vi "Call Asynchronous.vi"(8 "error in":errorcluster, 10 "Data In":variant, 11 "VI Path":path) -> (0 "error out":errorcluster)   [LabVIEW 2020]
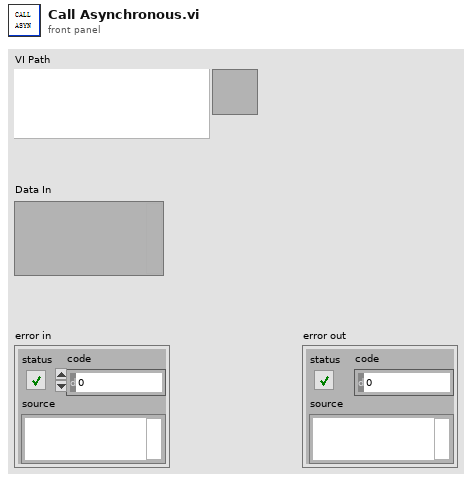
[diagram p1: front panel]
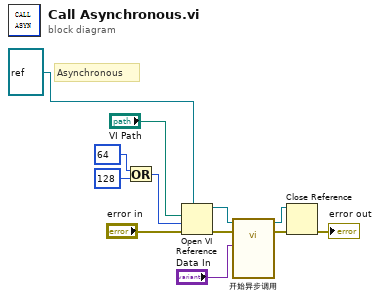
[diagram p0: block diagram]
diagram:
  # "Asynchronous"
  n1 = Or(x=64 ("选项"), y=128 ("选项")) -> (x .or. y?=w12:i32)
  n2 = Open VI Reference(type specifier VI Refnum (for type only)=refnum<vi> refnum, vi path="VI Path", options=w12, error in (no error)="error in") -> (vi reference=w11:refnum<vi>, error out=w10:errorcluster)  [unwired: 2 in]
  n3 = call-by-ref "开始异步调用"(reference=w11, error in=w10, "Data Interface"="Data In") -> (reference out=w3:refnum<vi>, error out=w2:errorcluster)  [unwired: 11 in]
  n4 = Close Reference(reference=w3, error in (no error)=w2) -> (error out=→"error out":errorcluster)
